vi "ExperimentSettings.vi"(4 "small?":bool, 5 "Experiment Settings id":u16, 6 "Enable":bool, 7 "Default Experiment Name":string caption="Please Enter Tags:", 8 "error in (no error)":errorcluster, 9 "current time":timestamp, 10 "default Experiment Description":string caption="Please Enter Experiment Description:", 11 "Default Group ID":u16(ring) items=["CCLDAS"=1, "LASP"=2, "CU"=3, "NLSI"=4, "LDEX"=5, "Heidelberg"=6]) -> (0 "error out":errorcluster, 3 "output cluster":T1)   [LabVIEW 2012]
uses:
  Public API/ExperimentSetting.ctl
  <vilib>/addons/database/NI_Database_API.lvlib
panel:
  in  "ExperimentSetting":T1
  # "Experiment Settings"
  # "Experiment Settings"
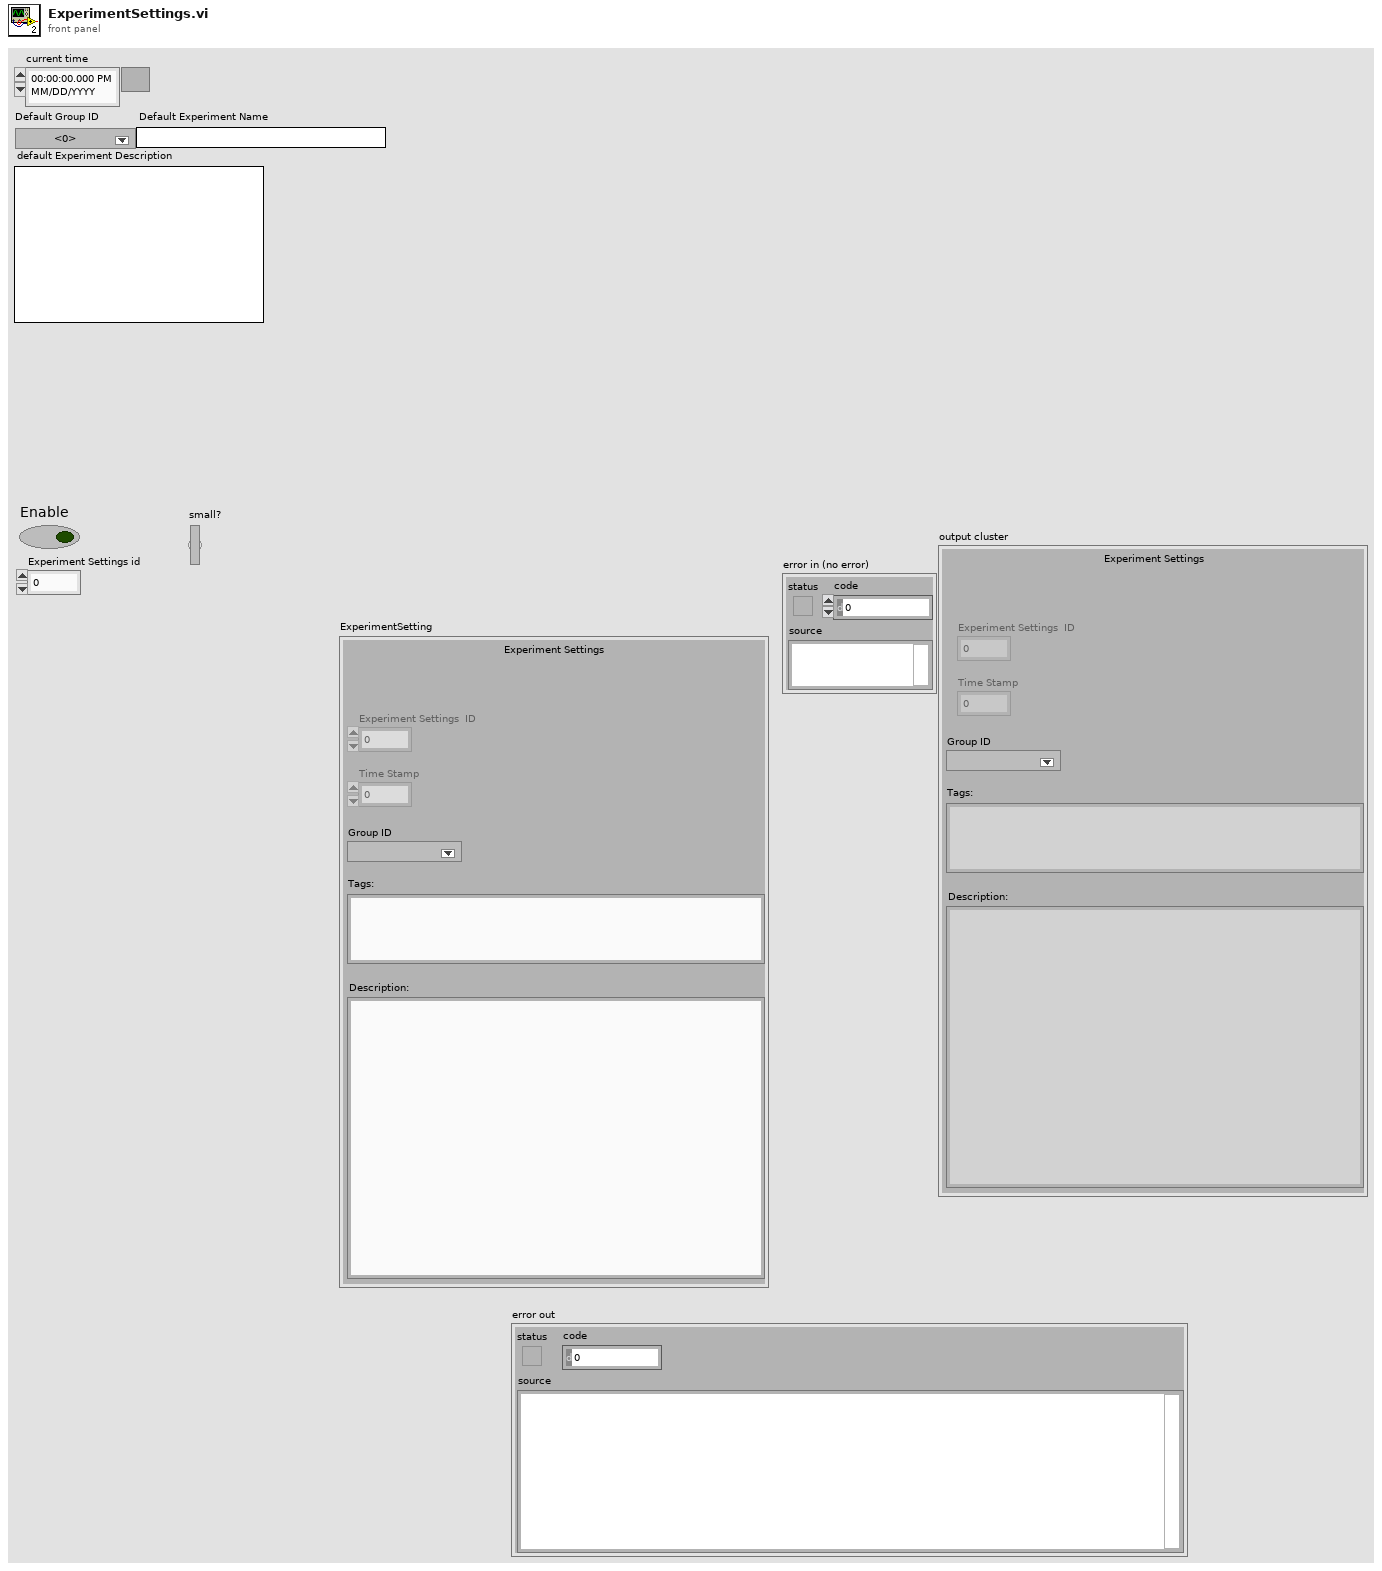
[diagram p1: front panel]
types:
  T1 = typedef "ExperimentSetting.ctl" = cluster{"Experiment Settings  ID":i64, "Time Stamp":i64, "Group ID":i32, "Tags:":string, "Description:":string}
  T2 = cluster{"Please Enter Tags:":string, "Please Enter Experiment Description:":string, "Default Group ID":i32}
  T3 = typedef "NI_Database_API.lvlib/Conn ObjectReference.ctl" = refnum<k1>
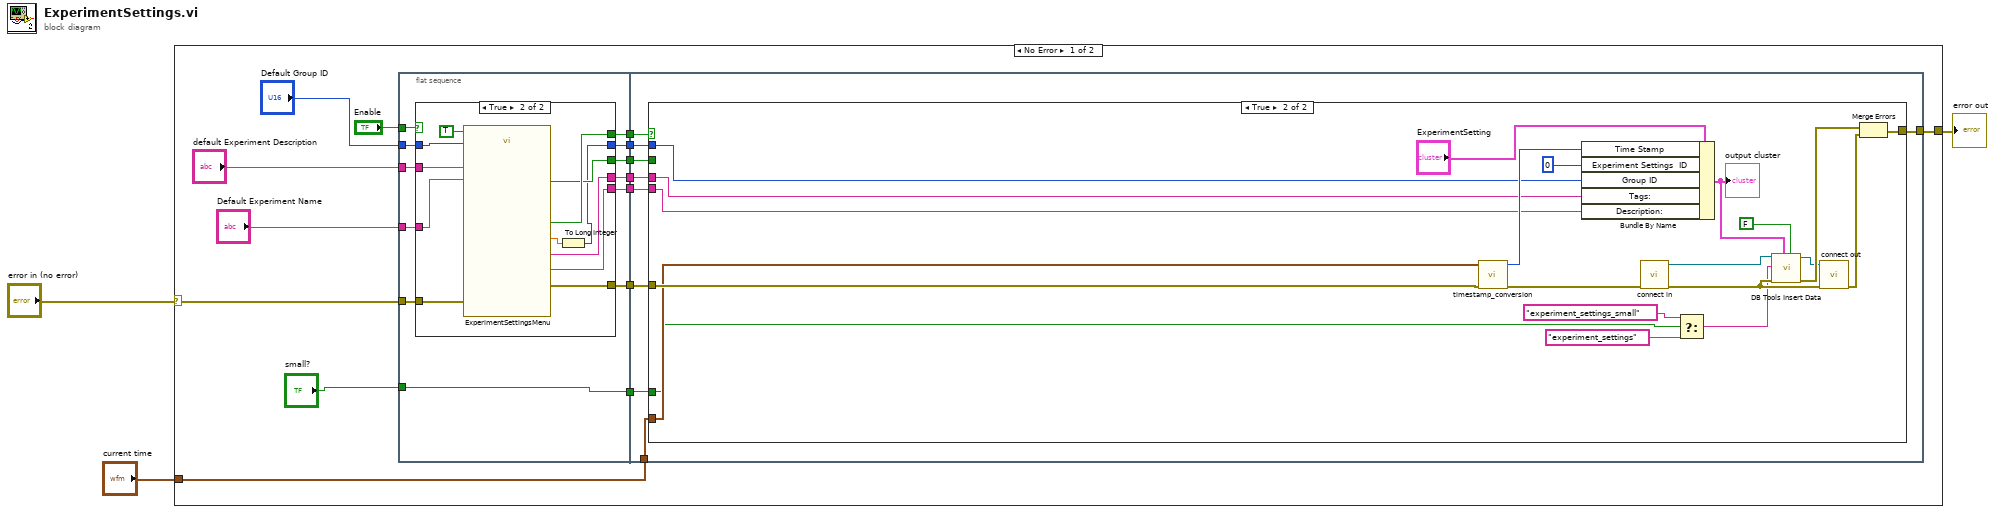
[diagram p0: block diagram]
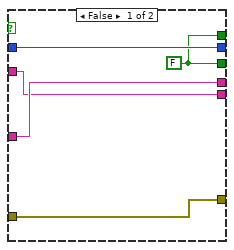
[diagram p2: hidden frame]
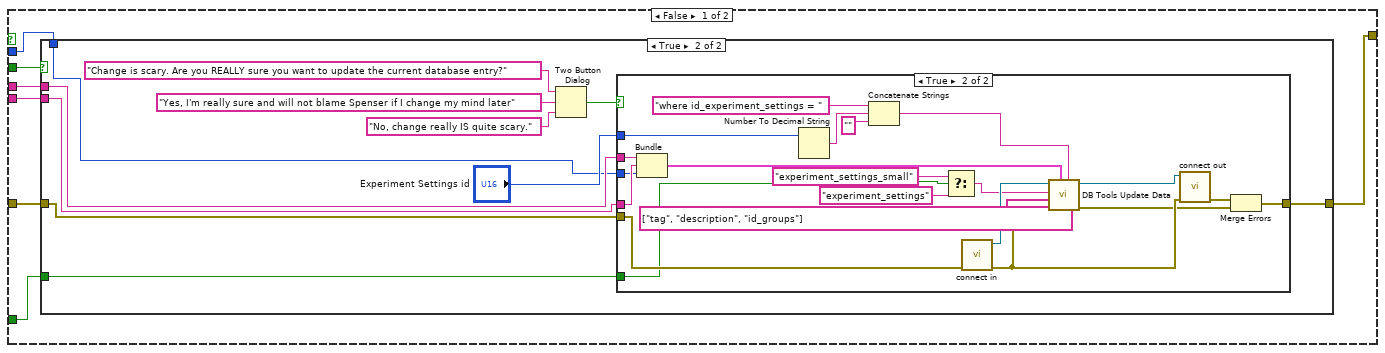
[diagram p3: hidden frame]
diagram:
  n1 = case shown="No Error" "error in (no error)" {
    selector: "error in (no error)" -> [w18 w119]
    tunnel: [w13 w119] -> w2
    tunnel: "current time" -> [w8 _]
    frame No Error {
      n2 = flat-sequence {
        tunnel: w18 -> [w30]
        tunnel: [w29] -> w17
        tunnel: [w28] -> w16
        tunnel: [w27] -> w15
        tunnel: [w26] -> w14
        tunnel: "Default Group ID" -> [w20]
        tunnel: "default Experiment Description" -> [w25]
        tunnel: "Default Experiment Name" -> [w24]
        tunnel: [w23] -> w9
        tunnel: "Enable" -> [w22]
        tunnel: [w21] -> w6
        tunnel: [w19] -> w5
        tunnel: "small?" -> [w19]
        tunnel: w17 -> [w56]
        tunnel: w16 -> [w55]
        tunnel: w15 -> [w54]
        tunnel: w14 -> [w53]
        tunnel: [w52] -> w13
        tunnel: w9 -> [w51]
        tunnel: w8 -> [w50]
        tunnel: w6 -> [w49]
        tunnel: w5 -> [w48]
        frame #0 {
          n3 = case shown="True" w22 {
            tunnel: w30 -> [w32 w47]
            tunnel: [w32 w46] -> w29
            tunnel: [w33 w45] -> w28
            tunnel: [w34 w44] -> w27
            tunnel: [w35 w36] -> w26
            tunnel: w20 -> [w35 w43]
            tunnel: w25 -> [w33 w42]
            tunnel: w24 -> [w34 w41]
            tunnel: [w31 w39] -> w23
            tunnel: [w31 w38] -> w21
            frame False {
              w31 = FALSE ("Cancel 2")
            }
            frame True {
              n4 = call "ExperimentSettingsMenu.vi"("Enable"=TRUE, "Default Group ID"=w43, "error in (no error)"=w47, "Default Experiment Name"=w41, "default Experiment Description"=w42) -> ("Update"=w38:bool, "Please Enter Experiment Description:"=w45:string, "Please Enter Tags:"=w44:string, "Please Enter Group ID"=w37:dbl, "New"=w39:bool, "error out"=w46:errorcluster)  [unwired: 8 in, 1 out]
              n5 = To Long Integer(number=w37) -> (32bit integer=w36:i32)
            }
          }
        }
        frame #1 {
          n6 = case shown="True" w51 {
            tunnel: w56 -> [w63 w107]
            tunnel: w55 -> [w60 w106]
            tunnel: w54 -> [w61 w105]
            tunnel: w53 -> [w58 w104]
            tunnel: [w62 w103] -> w52
            tunnel: w50 -> [_ w102]
            tunnel: w49 -> [w59 _]
            tunnel: w48 -> [w57 w99]
            frame False {
              n7 = case shown="True" w59 {
                tunnel: w63 -> [w64 w75]
                tunnel: [w64 w74] -> w62
                tunnel: w61 -> [_ w73]
                tunnel: w60 -> [_ w72]
                tunnel: w58 -> [_ w66]
                tunnel: w57 -> [_ w65]
                frame False {
                }
                frame True {
                  n8 = Two Button Dialog(message="Change is scary. Are you REALLY sure you want to update the current database entry?", 1:"No, change really IS quite scary." ("F button name (\"Cancel\")"), 2:"Yes, I'm really sure and will not blame Spenser if I change my mind later" ("T button name (\"OK\")")) -> (T button?=w70:bool)
                  n9 = case shown="True" w70 {
                    tunnel: w75 -> [w76 w83]
                    tunnel: [w76 w86] -> w74
                    tunnel: w73 -> [_ w92]
                    tunnel: w72 -> [_ w91]
                    tunnel: "Experiment Settings id" -> [_ w94]
                    tunnel: w66 -> [_ w81]
                    tunnel: w65 -> [_ w79]
                    frame False {
                    }
                    frame True {
                      n10 = Bundle("Please Enter Tags:"=w92, "Please Enter Experiment Description:"=w91, "Default Group ID"=w81) -> (w90:T2)  [unwired: 1 in]
                      n11 = Number To Decimal String(number=w94) -> (decimal integer string=w96:string)  [unwired: 1 in]
                      n12 = Concatenate Strings("where id_experiment_settings = " ("condition"), w96, "" ("string")) -> (w93:string)
                      n13 = Select(t="experiment_settings_small" ("table"), s=w79, f="experiment_settings" ("table")) -> (s? t:f=w77:string)
                      n14 = call "connect in.vi"("error in (no error)"=w83) -> ("error out"=w89:errorcluster, "Database Connection"=w87:T3)  [unwired: 6 in, 1 out]
                      n15 = call <vilib>:"DB Tools Update Data.vi"("condition"=w93, "data"=w90, "error in (no error)"=w89, "columns"=string[] ["tag", "description", "id_groups"], "table"=w77, "connection reference"=w87) -> ("error out"=w84:errorcluster, "connection reference out"=w88:T3)  [unwired: 4 in]
                      n16 = call "connect out.vi"("error in (no error)"=w89, "connection reference"=w88) -> ("error out"=w85:errorcluster)  [unwired: 9 in]
                      n17 = Merge Errors(w85, w84) -> (w86:errorcluster)
                    }
                  }
                }
              }
            }
            frame True {
              n18 = call "timestamp_conversion.vi"("error in (no error)"=w107, "Time Stamp"=w102) -> ("error out"=w117:errorcluster, "Integer Time"=w115:i64)  [unwired: 7 in]
              n19 = Bundle By Name(cluster="ExperimentSetting", "Time Stamp"=w115, "Experiment Settings  ID"=i64 0, "Group ID"=w104, "Tags:"=w105, "Description:"=w106) -> (w118:T1)
              "output cluster" <- w118
              n20 = call "connect in.vi"("error in (no error)"=w117) -> ("error out"=w112:errorcluster, "Database Connection"=w108:T3)  [unwired: 6 in, 1 out]
              n21 = Select(t="experiment_settings_small" ("table"), s=w99, f="experiment_settings" ("table")) -> (s? t:f=w100:string)
              n22 = call <vilib>:"DB Tools Insert Data.vi"("create table? (F)"=FALSE, "data"=w118, "error in (no error)"=w112, "table"=w100, "connection reference"=w108) -> ("error out"=w111:errorcluster, "connection reference out"=w110:T3)  [unwired: 5 in]
              n23 = call "connect out.vi"("error in (no error)"=w112, "connection reference"=w110) -> ("error out"=w113:errorcluster)  [unwired: 9 in]
              n24 = Merge Errors(w111, w113) -> (w103:errorcluster)
            }
          }
        }
      }
    }
    frame Error {
    }
  }
  "error out" <- w2
